vi "Get Custom Route Properties.vi"(8 "error in (no error)":errorcluster, 11 "Item Ref in":T3 format="%.0x") -> (0 "error out":errorcluster, 2 "Routes":T1, 3 "Item Ref out":T3 format="%.0x")   [LabVIEW 2019, in "NI Synchronization System Explorer.lvlib"]
uses:
  NI Synchronization System Explorer.lvlib
  <vilib>/NI VeriStand/Custom Device API/Custom Device Item Ref.ctl
  Shared/Routes.ctl
  Shared/Route.ctl
  Shared/Constants.vi
  <vilib>/NI VeriStand/Custom Device API/Get Item Property (String).vi
  <vilib>/NI VeriStand/Custom Device API/Custom Device API.lvlib
  Shared/NI Synchronization Shared.lvlib
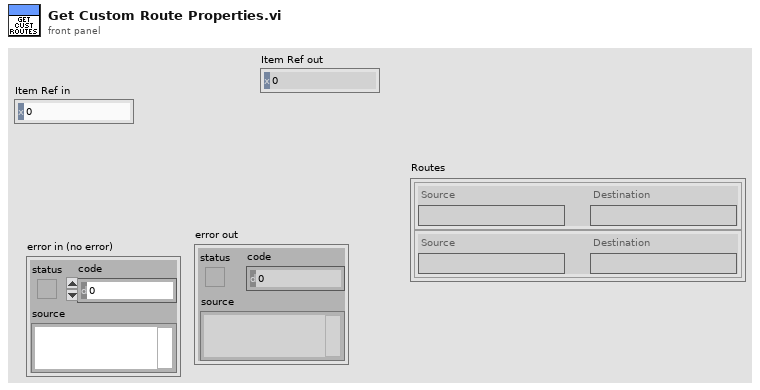
[diagram p1: front panel]
types:
  T1 = typedef "NI Synchronization Shared.lvlib/Routes.ctl" = T2[]
  T2 = typedef "NI Synchronization Shared.lvlib/Route.ctl" = cluster{"Source":string, "Destination":string}
  T3 = typedef "Custom Device API.lvlib/Custom Device Item Ref.ctl" = u64
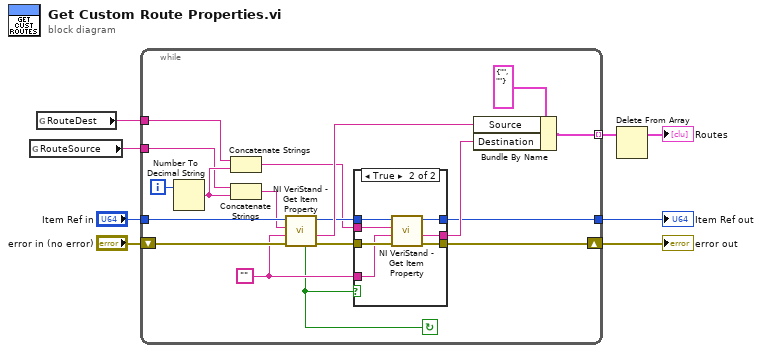
[diagram p0: block diagram]
diagram:
  n1 = global read "Constants.vi" "RouteSource"() -> (w6:string)
  n2 = global read "Constants.vi" "RouteDest"() -> (w5:string)
  n3 = while {
    shift-right: [w12] -> w3
    shift-left: "error in (no error)" -> [w26]
    tunnel: "Item Ref in" -> [w25]
    tunnel: w6 -> [w17]
    tunnel: w5 -> [w16]
    tunnel: [w11] -> w4
    tunnel: [w9] -> w2 mode=indexing
    i -> [w24]
    stop <- w10 continue-if-true
    w13 = ""
    n4 = Number To Decimal String(number=w24) -> (decimal integer string=w18:string)  [unwired: 1 in]
    n5 = Concatenate Strings(w16, w18) -> (w15:string)
    n6 = Concatenate Strings(w17, w18) -> (w23:string)
    n7 = call-poly <vilib>:"NI VeriStand - Get Item Property.vi"("error in (no error)"=w26, "Default Value"=w13, "Property Name"=w23, "Item Ref in"=w25) -> ("error out"=w20:errorcluster, "Value"=w21:string, "Item Ref out"=w19:T3, "Found?"=w10:bool)  [unwired: 4 in]
    n8 = case shown="True" w10 {
      tunnel: w20 -> [w28 w36]
      tunnel: w19 -> [w29 w35]
      tunnel: w15 -> [_ w34]
      tunnel: [w27 w33] -> w14
      tunnel: w13 -> [w27 w32]
      tunnel: [w28 w31] -> w12
      tunnel: [w29 w30] -> w11
      frame False {
      }
      frame True {
        n9 = call-poly <vilib>:"NI VeriStand - Get Item Property.vi"("error in (no error)"=w36, "Default Value"=w32, "Property Name"=w34, "Item Ref in"=w35) -> ("error out"=w31:errorcluster, "Value"=w33:string, "Item Ref out"=w30:T3)  [unwired: 4 in, 1 out]
      }
    }
    n10 = Bundle By Name(cluster=T2 {"Source"="", "Destination"=""} ("Route"), "Source"=w21, "Destination"=w14) -> (w9:T2)
  }
  "error out" <- w3
  "Item Ref out" <- w4
  n11 = Delete From Array(array=w2) -> (array with subset deleted=→"Routes":T2[])  [unwired: 2 in, 1 out]
